vi "VRM_parse_status.vi"(11 "PSU Act Stat":T1) -> (3 "String":string)   [LabVIEW 2016]
uses:
  <instrlib>/Mercury iXX/Public/Libraries/Magnet/Controls/PSU Actions.ctl
  <instrlib>/Mercury iXX/Public/Libraries/Magnet.lvlib
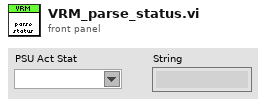
[diagram p1: front panel]
types:
  T1 = typedef "Mercury iXX.lvlib/Magnet.lvlib/PSU Actions.ctl" = string
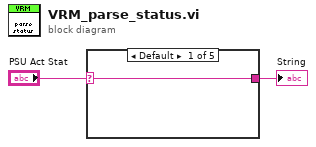
[diagram p0: block diagram]
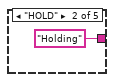
[diagram p2: hidden frame]
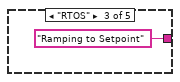
[diagram p3: hidden frame]
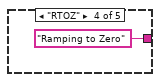
[diagram p4: hidden frame]
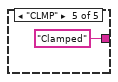
[diagram p5: hidden frame]
diagram:
  n1 = case shown="Default" "PSU Act Stat" {
    selector: "PSU Act Stat" -> [w3 _ _ _ _]
    tunnel: [w3 "Holding" "Ramping to Setpoint" "Ramping to Zero" "Clamped"] -> w1
    frame Default {
    }
    frame "HOLD" {
    }
    frame "RTOS" {
    }
    frame "RTOZ" {
    }
    frame "CLMP" {
    }
  }
  "String" <- w1
